vi "Find Available Files.vi"(8 "error in (no error)":errorcluster, 11 "components directory":path) -> (0 "error out":errorcluster, 3 "paths":path[](array[path]))   [LabVIEW 2020, in "DSF System Explorer.lvlib"]
uses:
  DSF System Explorer.lvlib
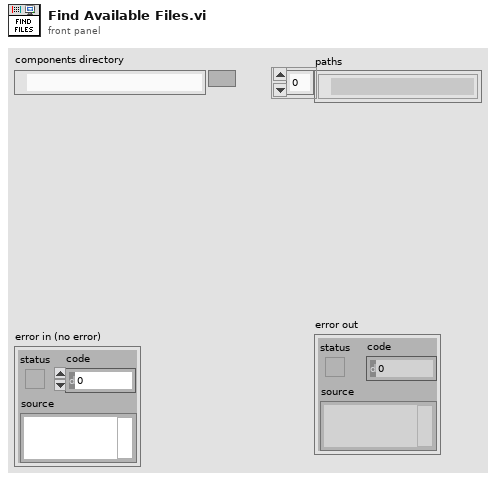
[diagram p1: front panel]
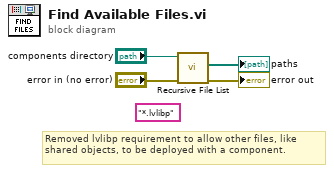
[diagram p0: block diagram]
diagram:
  (unwired) "*.lvlibp" ("pattern")
  # "Removed lvlibp requirement to allow other files, like shared objects, to be deployed with a component."
  n1 = call <vilib>:"Recursive File List.vi"("error in (no error)"="error in (no error)", "Folder Path"="components directory") -> ("error out"=→"error out":errorcluster, "All Files in Dir"=→"paths":path[])  [unwired: 5 in, 3 out]
